vi "Build Charting Config.vi"(8 "error in (no error)":errorcluster, 11 "Historian Charting Manager in":refnum<class "Historian Charting Manager.lvclass">) -> (0 "error out":errorcluster, 2 "Charting Config Value":refnum<class "Charting Config Value.lvclass">, 3 "Historian Charting Manager out":refnum<class "Historian Charting Manager.lvclass">)   [LabVIEW 2020, in "VolatusGUI.lvlib" / "Historian Charting Manager.lvclass"]
uses:
  Historian Charting Manager.lvclass
  Historian Charting Manager.lvclass/Historian Charting Manager.ctl
  JSON Chart Group.ctl
  VolatusGUI.lvlib
  JSON Plot Config.ctl
  JSON Plot Group.ctl
  JSON Charting Config.ctl
  Charting Config Value/Charting Config Value.lvclass
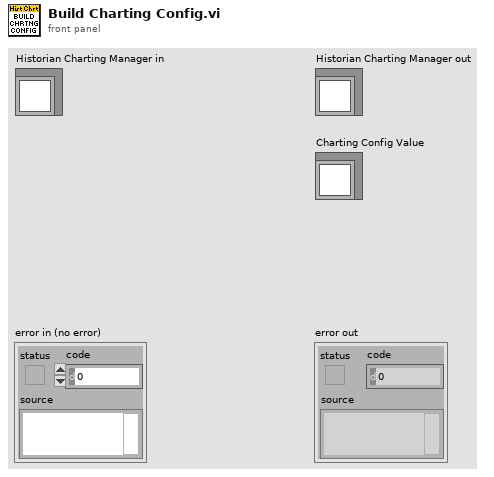
[diagram p1: front panel]
types:
  T1 = typedef "VolatusGUI.lvlib/JSON Charting Config.ctl" = cluster{"ChartGroups":T2[], "PlotGroups":T3[]}
  T2 = typedef "VolatusGUI.lvlib/JSON Chart Group.ctl" = cluster{"Name":string, "PlotGroups":string[]}
  T3 = typedef "VolatusGUI.lvlib/JSON Plot Group.ctl" = cluster{"Name":string, "Chart":cluster{"X-Axis":string, "X-Channel":string, "Now":bool, "Time":string, "SwapAxes":bool}, "Plots":T4[]}
  T4 = typedef "VolatusGUI.lvlib/JSON Plot Config.ctl" = cluster{"Channel":string, "Visible":bool, "Color":string, "Scale":string}
  T5 = typedef "VolatusGUI.lvlib/Historian Charting Manager.lvclass/Plot Group Config.ctl" = cluster{"Name":string, "X-Axis Type":T6, "X-Axis Channel":string, "Plots":T7[], "Lock Now":bool, "Time":string, "Swap Axes":bool}
  T6 = typedef "VolatusGUI.lvlib/Historian Charting Manager.lvclass/X-Axis Type.ctl" = enum16{"Time", "Channel"}
  T7 = typedef "VolatusGUI.lvlib/Historian Charting Manager.lvclass/Plot Config.ctl" = cluster{"Channel":string, "Visible":bool, "Color":u32, "Scale":T8}
  T8 = typedef "VolatusGUI.lvlib/Historian Charting Manager.lvclass/Scale.ctl" = enum16{"Left", "Right"}
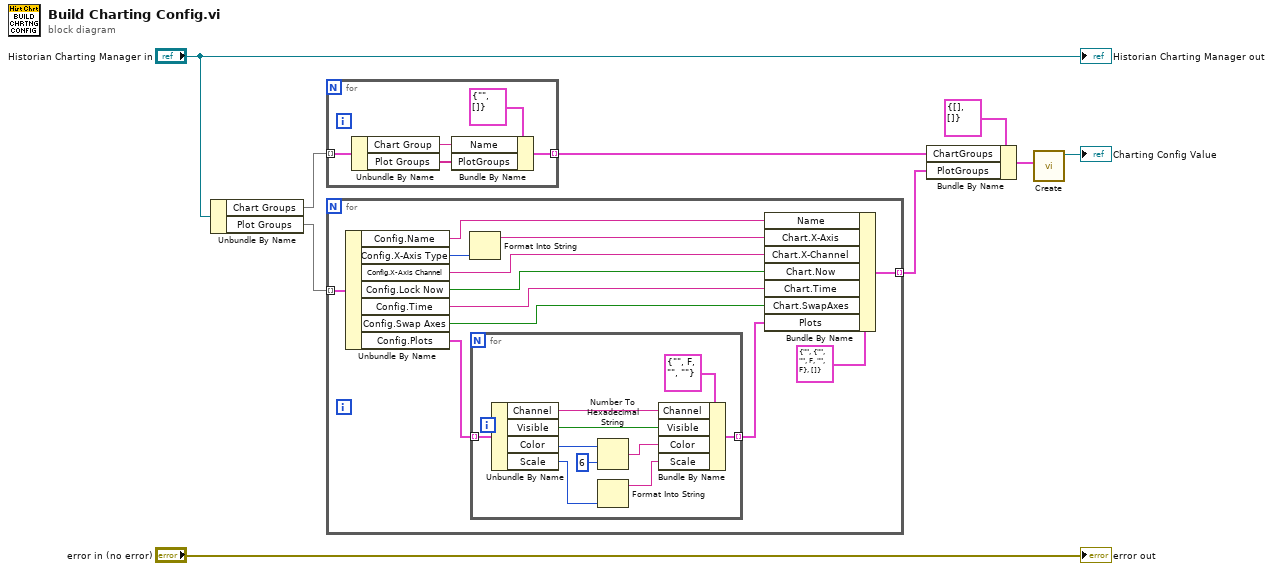
[diagram p0: block diagram]
diagram:
  n1 = Unbundle By Name("Historian Charting Manager in") -> ("Chart Groups"=w7:map{string, string[]}, "Plot Groups"=w6:map{string, T5})
  n2 = for {
    tunnel: w7 -> [w14] mode=indexing
    tunnel: [w10] -> w4 mode=indexing
    n3 = Unbundle By Name(w14) -> ("Chart Group"=w12:string, "Plot Groups"=w11:string[])
    n4 = Bundle By Name(cluster=T2 {"Name"="", "PlotGroups"=[]} ("JSON Chart Group"), "Name"=w12, "PlotGroups"=w11) -> (w10:T2)
  }
  n5 = for {
    tunnel: w6 -> [w26] mode=indexing
    tunnel: [w15] -> w3 mode=indexing
    n6 = Unbundle By Name(w26) -> ("Config.Name"=w24:string, "Config.X-Axis Type"=w23:T6, "Config.X-Axis Channel"=w21:string, "Config.Lock Now"=w20:bool, "Config.Time"=w19:string, "Config.Swap Axes"=w18:bool, "Config.Plots"=w17:T7[])
    n7 = Format Into String(w23) -> (resulting string=w22:string)  [unwired: 3 in, 1 out]
    n8 = for {
      tunnel: w17 -> [w36] mode=indexing
      tunnel: [w32] -> w16 mode=indexing
      n9 = Unbundle By Name(w36) -> ("Channel"=w34:string, "Visible"=w33:bool, "Color"=w31:u32, "Scale"=w29:T8)
      n10 = Number To Hexadecimal String(1:i16 6 ("width (-)"), 2:w31) -> (0:w27:string)
      n11 = Format Into String(w29) -> (resulting string=w28:string)  [unwired: 3 in, 1 out]
      n12 = Bundle By Name(cluster=T4 {"Channel"="", "Visible"=FALSE, "Color"="", "Scale"=""} ("Plot Config"), "Channel"=w34, "Visible"=w33, "Color"=w27, "Scale"=w28) -> (w32:T4)
    }
    n13 = Bundle By Name(cluster=T3 {"Name"="", "Chart"={"X-Axis"="", "X-Channel"="", "Now"=FALSE, "Time"="", "SwapAxes"=FALSE}, "Plots"=[]} ("JSON Plot Group"), "Name"=w24, "Chart.X-Axis"=w22, "Chart.X-Channel"=w21, "Chart.Now"=w20, "Chart.Time"=w19, "Chart.SwapAxes"=w18, "Plots"=w16) -> (w15:T3)
  }
  n14 = Bundle By Name(cluster=T1 {"ChartGroups"=[], "PlotGroups"=[]} ("JSON Charting Config"), "ChartGroups"=w4, "PlotGroups"=w3) -> (w2:T1)
  n15 = call "Create.vi"("JSON Charting Config"=w2) -> ("Charting Config Value out"=→"Charting Config Value":refnum<class "Charting Config Value.lvclass">)  [unwired: 10 in]
  "error out" <- "error in (no error)"
  "Historian Charting Manager out" <- "Historian Charting Manager in"
